vi "LabVIEW_ArduinoControlsNoHeater.vi"() -> ()   [LabVIEW 2021]
uses:
  <vilib>/Instr/_visa.llb/VISA Configure Serial Port (Instr).vi
panel:
  out "Horz Distance":dbl[](graph)
  out "Vert Distance":dbl[](graph)
  in  "DRILL STOP":bool
  in  "Drill Speed Arduino 2.0 Write Stop":bool
  in  "Slow Down":bool
  in  "Speed Up":bool
  in  "Drill Speed Arduino 2 Write":refnum<visa-resource-name>
  in  "Stepper Arduino 1 Serial Read":refnum<visa-resource-name>
  out "Weight on Bit A1":dbl[](graph)
  out "Vertical Motor Speed A1":dbl[](graph)
  out "Data Packet Arduini 1 Matched":i32
  in  "Arduino 1.0 Read Stop":bool
  in  "Arduino 2.0 Read Stop":bool
  in  "Emergency Stop! 3":bool
  in  "Emergency Stop! 2":bool
  in  "GO DOWN 3":bool
  in  "GO DOWN 2":bool
  in  "GO UP 3":bool
  in  "GO UP 2":bool
  in  "MAX SPEED 3":bool
  in  "MAX SPEED 2":bool
  in  "SLOWEST SPEED 3":bool
  in  "SLOWEST SPEED 2":bool
  in  "Decellerate 3":bool
  in  "Decellerate 2":bool
  in  "Accelerate 3":bool
  in  "Accelerate 2":bool
  in  "Drill Speed Arduino 2 Serial Read":refnum<visa-resource-name>
  out "Data Packet Received":i32
  out "RPM":dbl[](graph)
  in  "GO UP":bool
  in  "GO DOWN":bool
  in  "MAX SPEED":bool
  in  "SLOWEST SPEED":bool
  out "System Amps A2":dbl[](graph)
  out "concatenated string":string
  in  "Arduino 1.0 Write Stop":bool
  in  "Emergency Stop!":bool
  in  "Decellerate":bool
  in  "Stepper Arduino 1 Write":refnum<visa-resource-name>
  in  "Accelerate":bool
  # "Drill Speed Controls"
  # "WINCH CONTROLS"
  # "VERTICAL STEPPER MOTOR CONTROLS"
  # "HORIZONTAL STEPPER MOTOR CONTROLS"
  # "-1 Means Not Found\nany value greater than 0 corresponds to the amount\nof matching characters found"
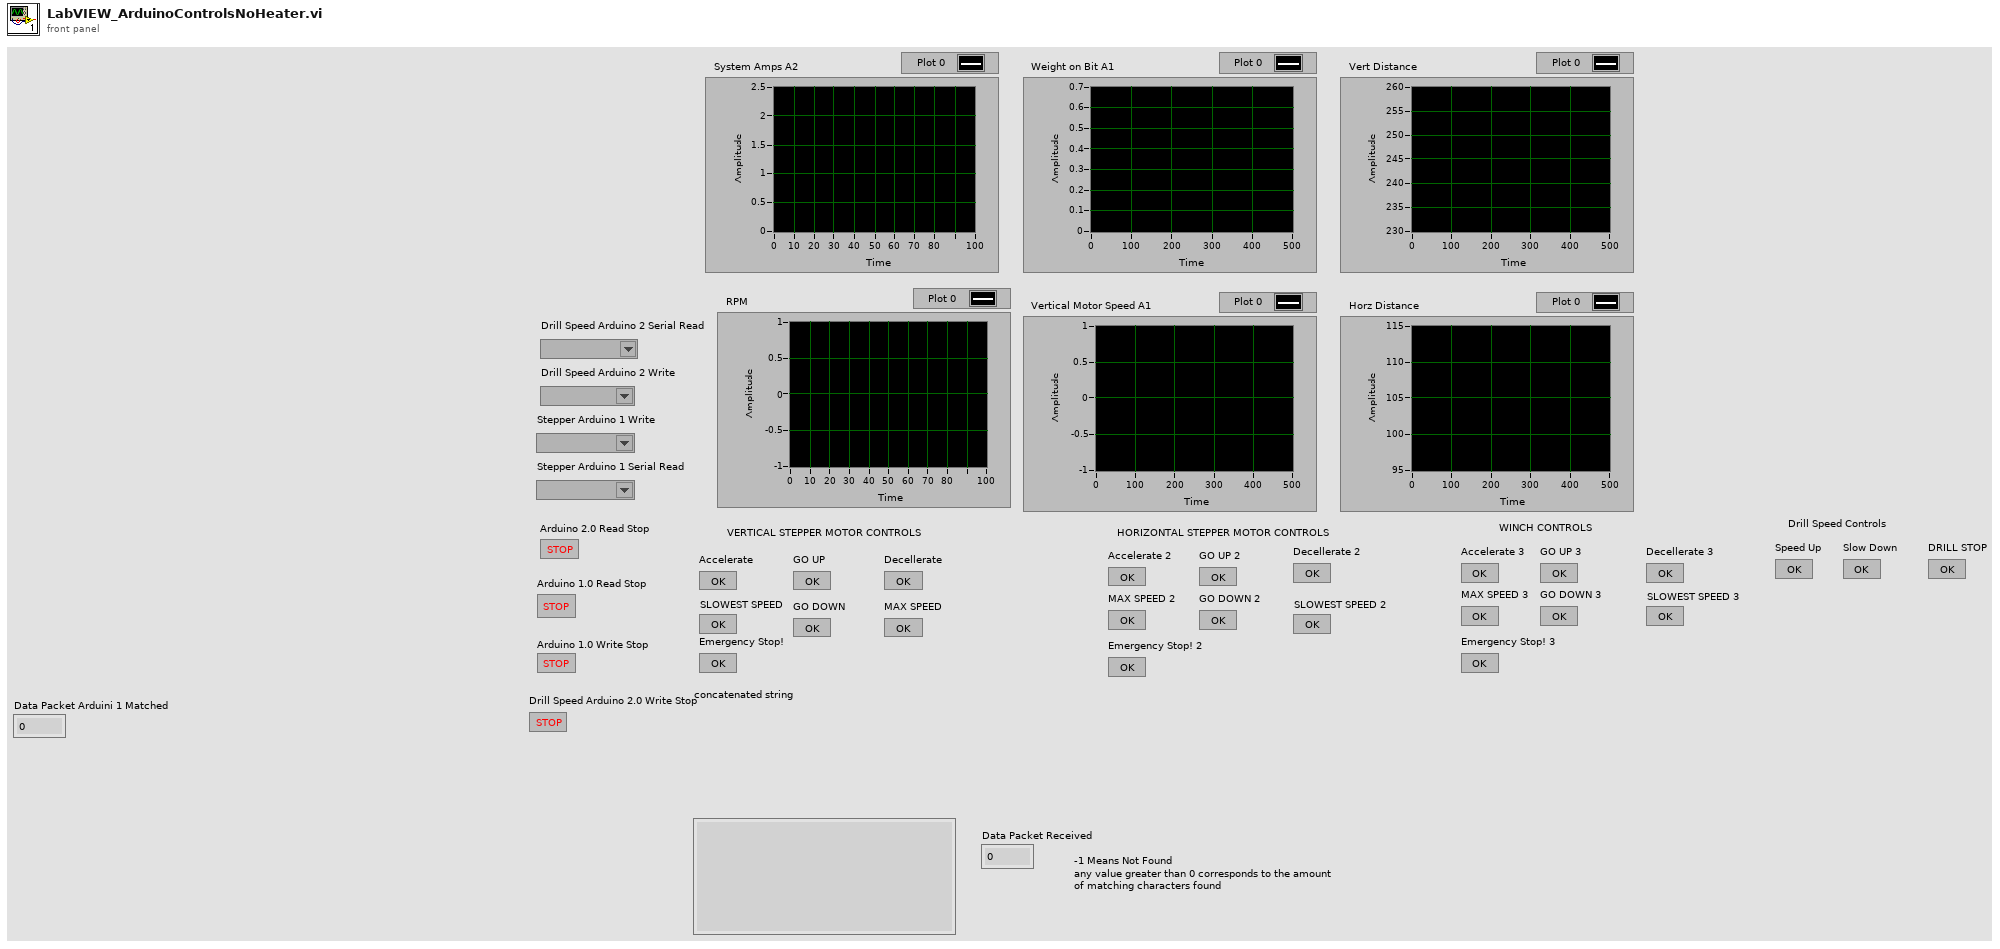
[diagram p1: front panel]
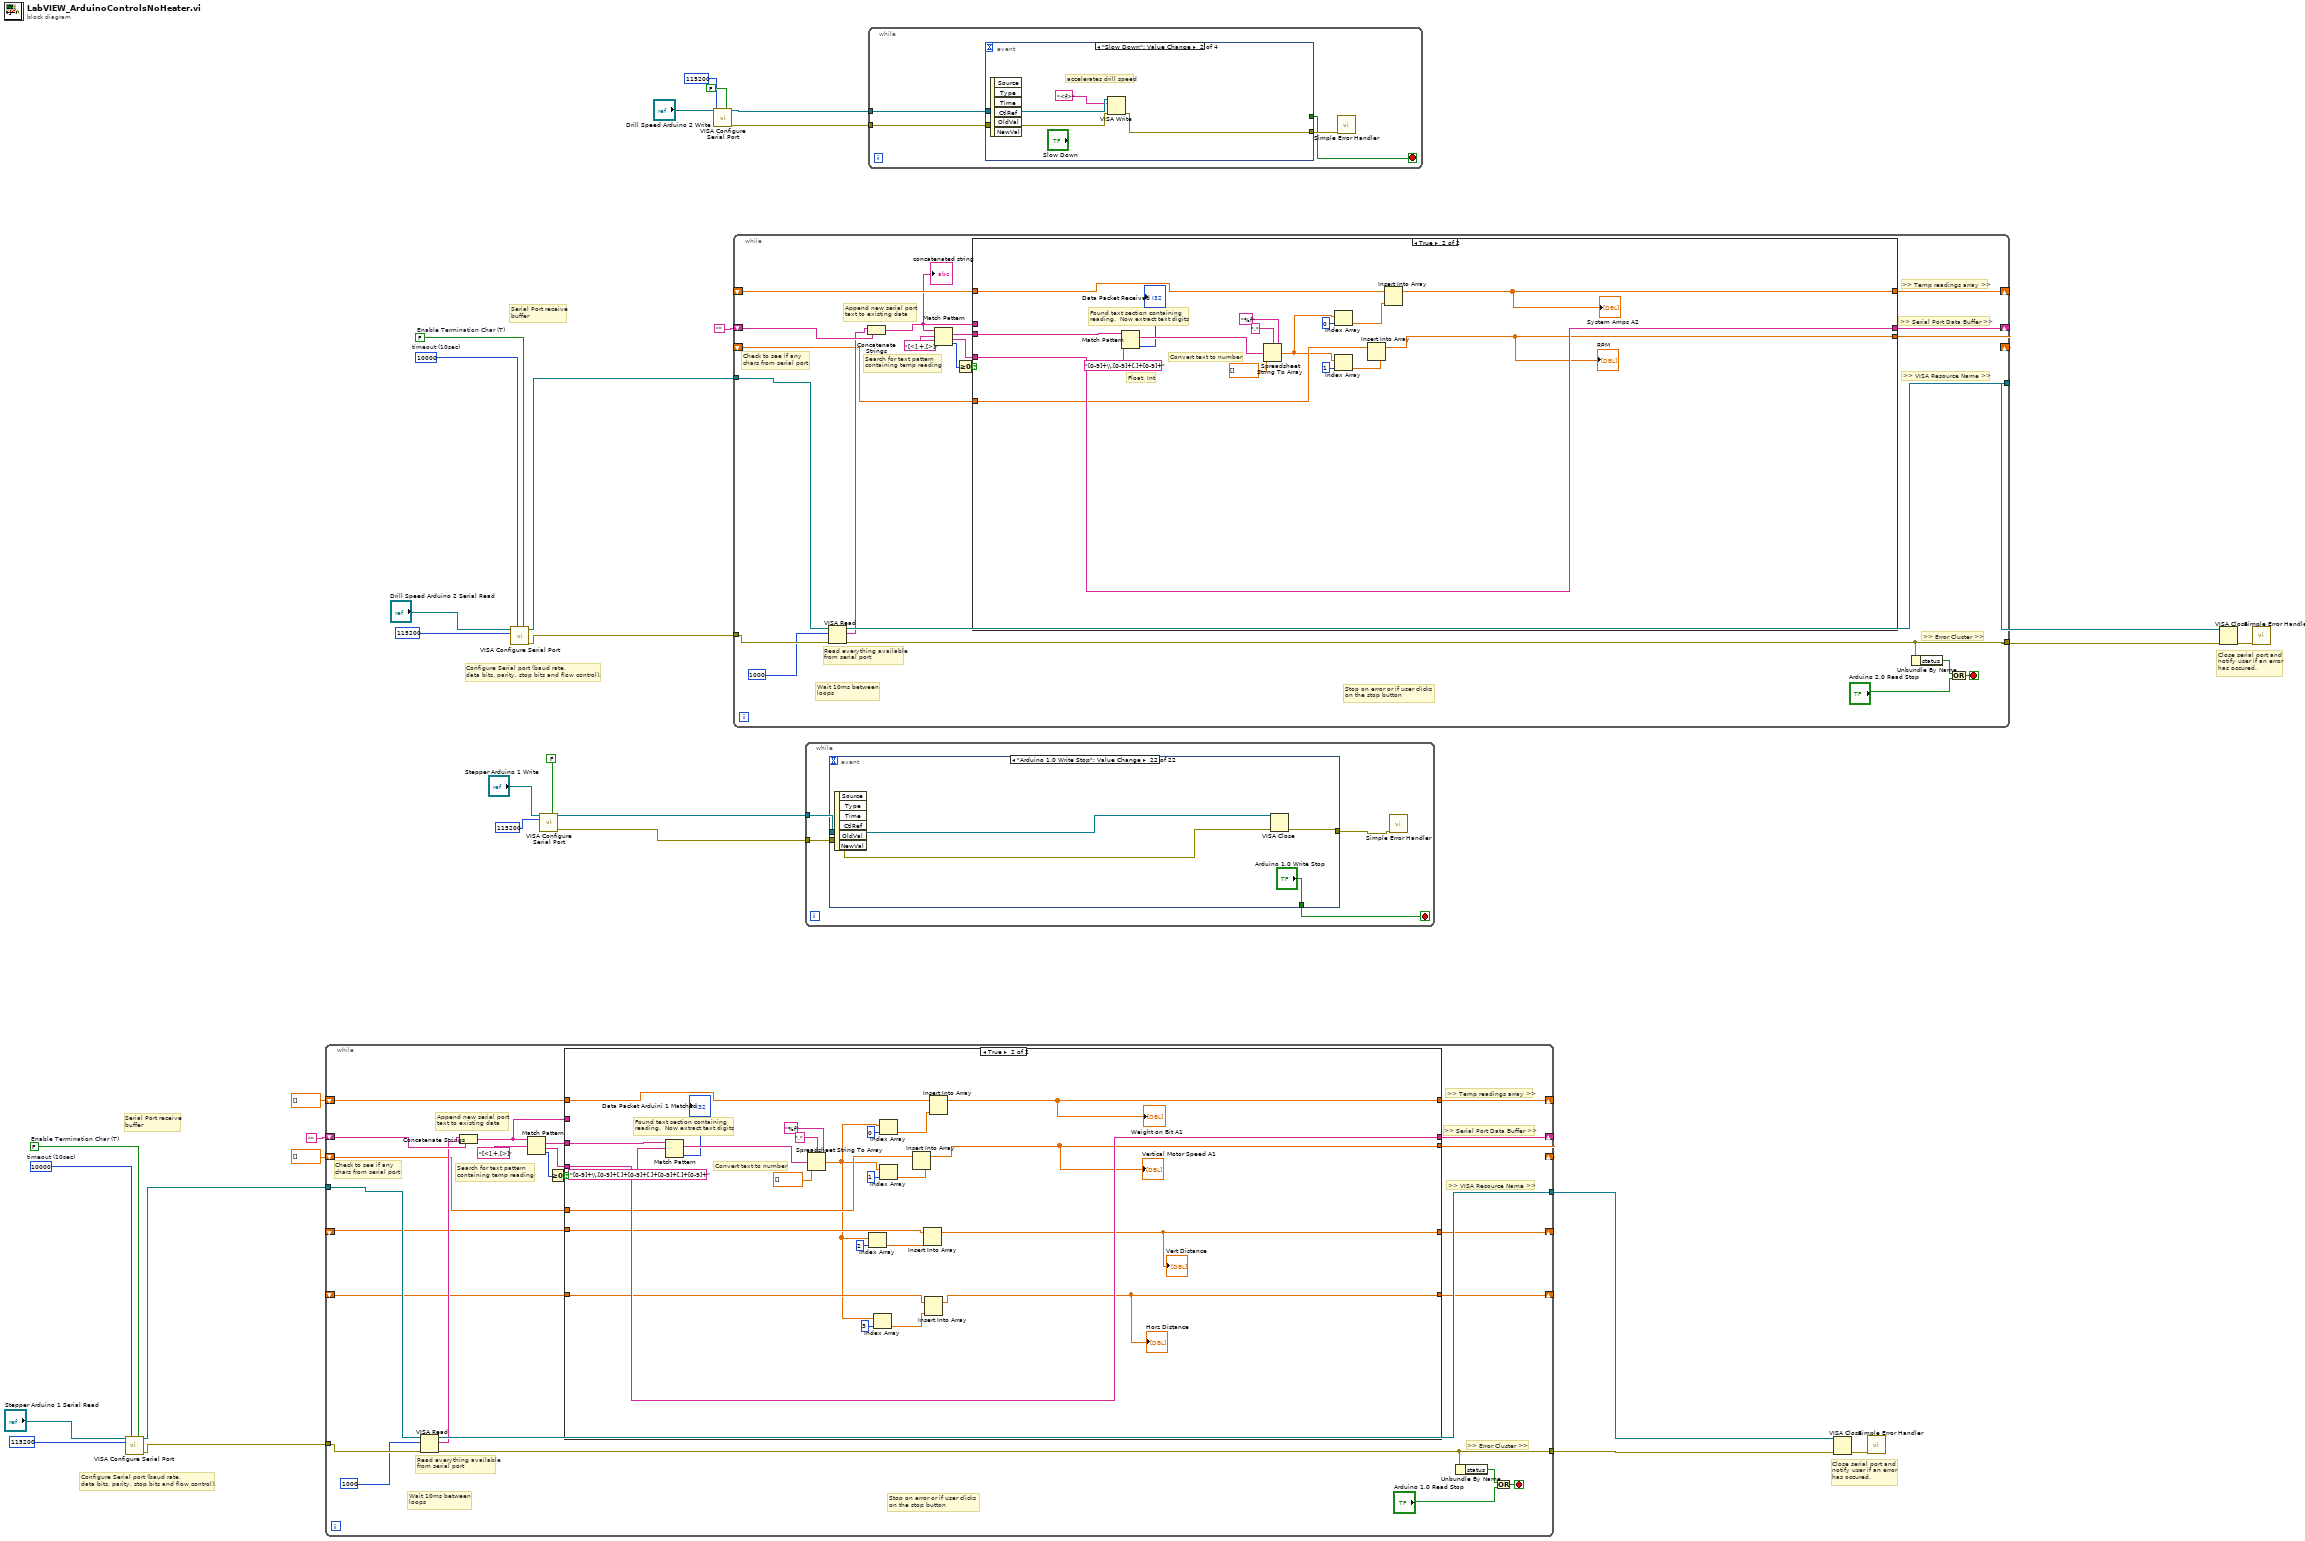
[diagram p0: block diagram]
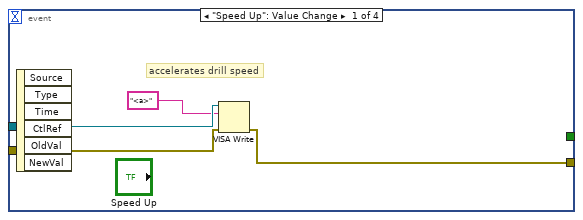
[diagram p2: hidden frame]
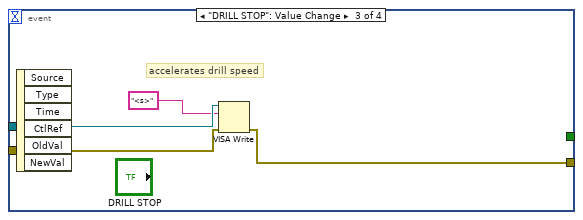
[diagram p3: hidden frame]
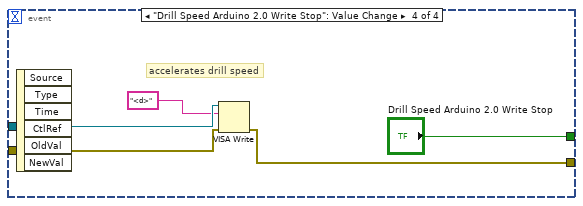
[diagram p4: hidden frame]
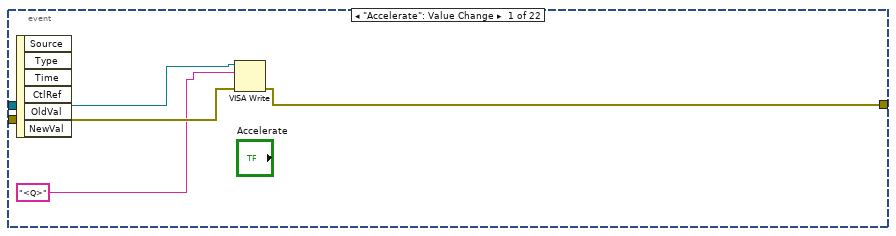
[diagram p7: hidden frame]
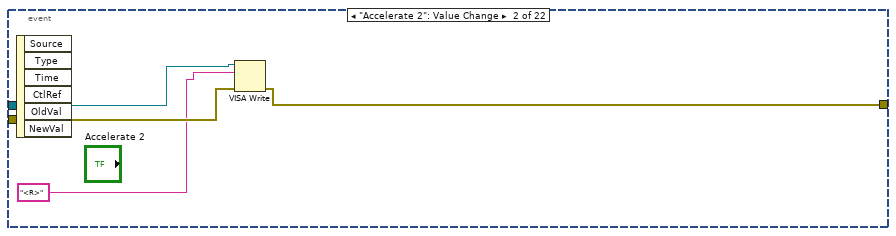
[diagram p8: hidden frame]
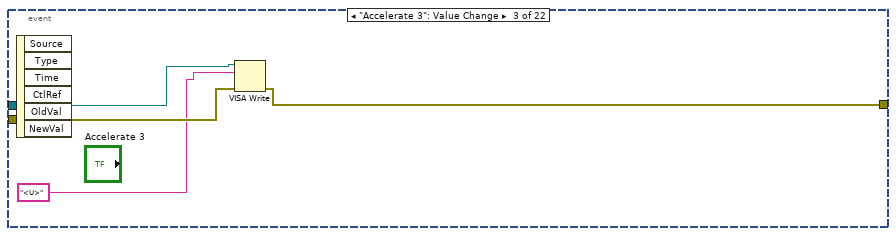
[diagram p9: hidden frame]
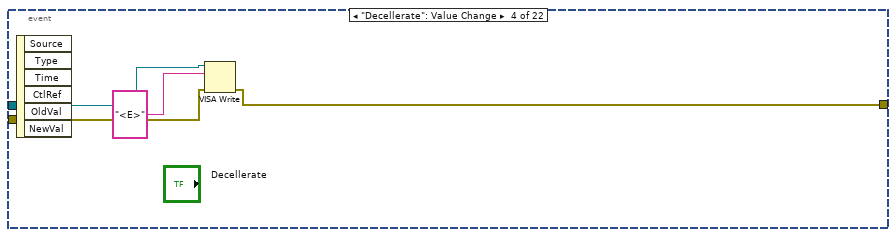
[diagram p10: hidden frame]
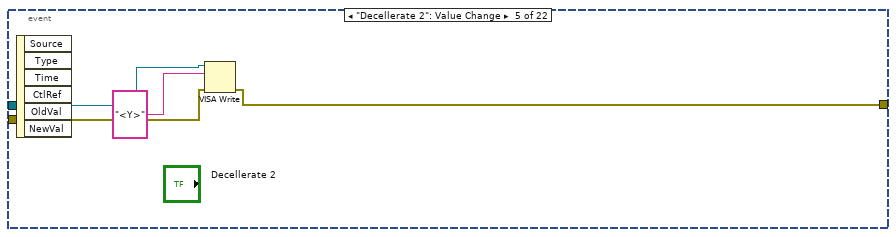
[diagram p11: hidden frame]
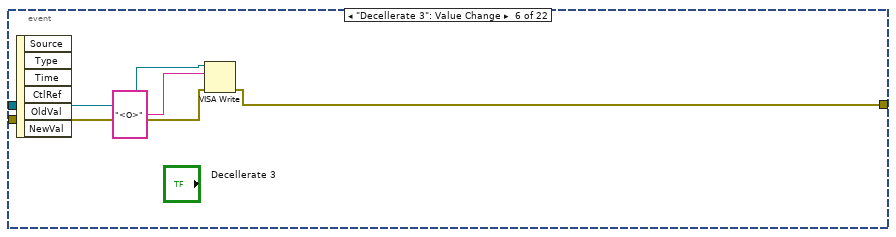
[diagram p12: hidden frame]
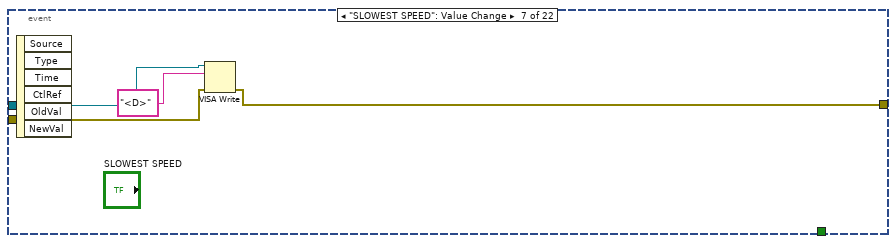
[diagram p13: hidden frame]
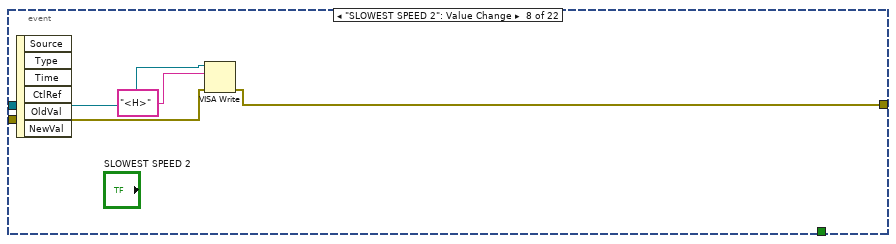
[diagram p14: hidden frame]
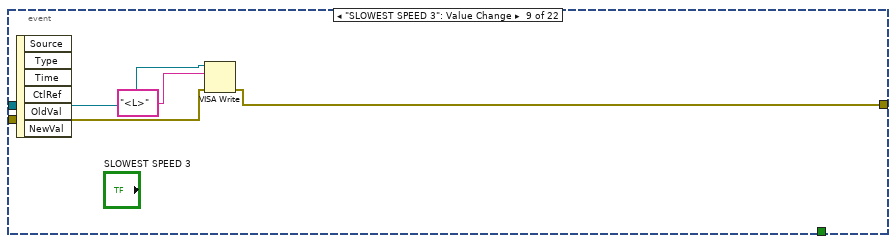
[diagram p15: hidden frame]
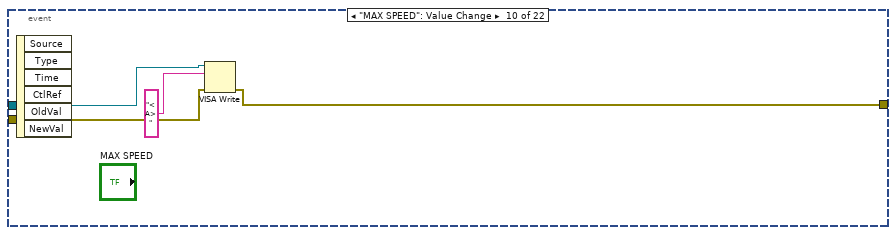
[diagram p16: hidden frame]
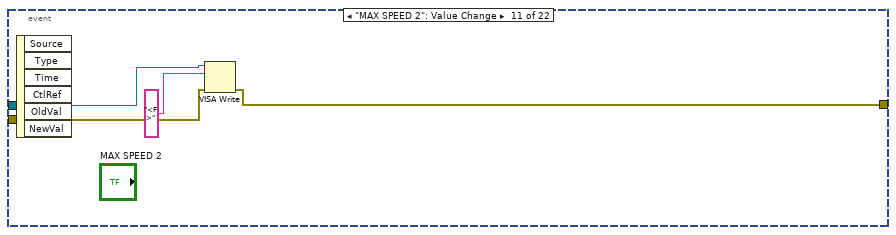
[diagram p17: hidden frame]
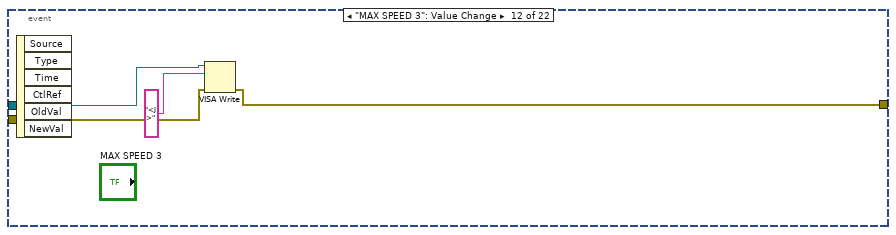
[diagram p18: hidden frame]
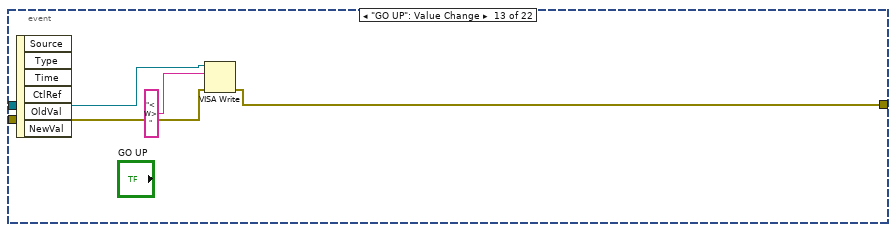
[diagram p19: hidden frame]
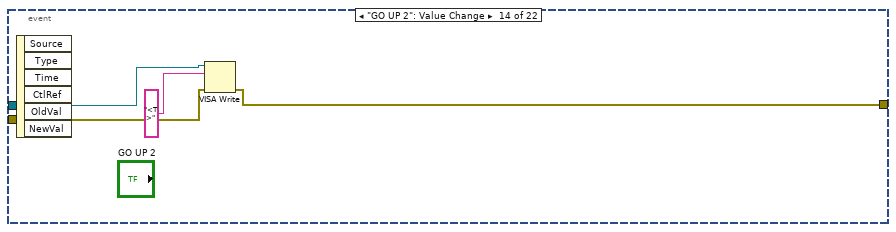
[diagram p20: hidden frame]
diagram:
  w13 = FALSE  # Enable Termination Char (T)
  w14 = u32 10000  # timeout (10sec)
  w24 = FALSE  # Enable Termination Char (T)
  w25 = u32 10000  # timeout (10sec)
  # "Close serial port and\nnotify user if an error\nhas occured."
  # "Serial Port receive\nbuffer"
  # "Configure Serial port (baud rate,\ndata bits, parity, stop bits and flow control)."
  # "Close serial port and\nnotify user if an error\nhas occured."
  # "Serial Port receive\nbuffer"
  # "Configure Serial port (baud rate,\ndata bits, parity, stop bits and flow control)."
  n1 = call-poly "VISA Configure Serial Port"("VISA resource name"="Stepper Arduino 1 Serial Read", "timeout (10sec)"=w14, "Enable Termination\nChar (T)"=w13, "baud rate (9600)"=u32 115200) -> ("VISA resource name out"=w10:refnum<visa-resource-name>, "error out"=w9:errorcluster)  [unwired: 10 in]
  n2 = while {
    tunnel: [w55] -> w17
    tunnel: [w57] -> w16
    shift-right: [w50] -> _
    shift-left: "" -> [w56]
    shift-right: [w52] -> _
    shift-left: dbl[] [] -> [w51]
    tunnel: w10 -> [w49]
    tunnel: w9 -> [w48]
    shift-right: [w40] -> _
    shift-left: dbl[] [] -> [w39]
    shift-right: [w35] -> _
    shift-left: _ -> [w36]
    shift-right: [w33] -> _
    shift-left: _ -> [w34]
    stop <- w54 stop-if-true
    # "Search for text pattern\ncontaining temp reading"
    # "Append new serial port\ntext to existing data"
    # "Read everything available\nfrom serial port"
    # "Wait 10ms between \nloops"
    # "Stop on error or if user clicks \non the stop button"
    # ">> Error Cluster >>"
    # ">> VISA Resource Name >>"
    # ">> Temp readings array >>"
    # ">> Serial Port Data Buffer >>"
    # "Check to see if any\nchars from serial port"
    n3 = VISA Read(VISA resource name=w49, byte count=u32 1000, error in (no error)=w48) -> (VISA resource name out=w57:refnum<visa-resource-name>, read buffer=w42:string, error out=w55:errorcluster)  [unwired: 1 out]
    n4 = Concatenate Strings(w42, w56) -> (w37:string)
    n5 = Match Pattern(string=w37, regular expression="[<].+.[>]") -> (match substring=w44:string, after substring=w43:string, offset past match=w46:i32)  [unwired: 1 in, 1 out]
    n6 = Greater Or Equal To 0?(x=w46) -> (x >= 0?=w45:bool)
    n7 = case shown="True" w45 {
      tunnel: w44 -> [_ w86]
      tunnel: w43 -> [_ w87]
      tunnel: [w60 w87] -> w50
      tunnel: [w62 w84] -> w52
      tunnel: w51 -> [w62 w72]
      tunnel: [w61 w75] -> w40
      tunnel: w39 -> [w61 w76]
      tunnel: w37 -> [w60 _]
      tunnel: w36 -> [w59 w70]
      tunnel: [w59 w68] -> w35
      tunnel: w34 -> [w58 w66]
      tunnel: [w58 w63] -> w33
      frame False {
        # "Did not find text pattern in the buffer.  Try again in the next loop after new data \nhas been received."
      }
      frame True {
        # "Convert text to number"
        # "Found text section containing \nreading.  Now extract text digits"
        n8 = Match Pattern(string=w86, regular expression="[0-9]+\\.[0-9]+[,]+[0-9]+[,]+[0-9]+[,]+[0-9]+") -> (match substring=w79:string, offset past match=→"Data Packet Arduini 1 Matched":i32)  [unwired: 1 in, 2 out]
        n9 = Spreadsheet String To Array(delimiter (Tab)=",", format string="%f", spreadsheet string=w79, array type (2D Dbl)=dbl[] []) -> (array=w65:dbl[])
        n10 = Index Array(array=w65, index=2) -> (element=w71:dbl)
        n11 = Index Array(array=w65, index=3) -> (element=w67:dbl)
        n12 = Index Array(array=w65, index=0 ("index (row)")) -> (element=w78:dbl)
        n13 = Index Array(array=w65, index=1 ("index (row)")) -> (element=w77:dbl)
        n14 = Insert Into Array(array=w76, new element=w77) -> (w75:dbl[])  [unwired: 1 in]
        "Vertical Motor Speed A1" <- w75
        n15 = Insert Into Array(array=w70, new element=w71) -> (w68:dbl[])  [unwired: 1 in]
        "Vert Distance" <- w68
        n16 = Insert Into Array(array=w66, new element=w67) -> (w63:dbl[])  [unwired: 1 in]
        "Horz Distance" <- w63
        n17 = Insert Into Array(array=w72, new element=w78) -> (w84:dbl[])  [unwired: 1 in]
        "Weight on Bit A1" <- w84
      }
    }
    n18 = Unbundle By Name(w55) -> ("status"=w53:bool)
    n19 = Or(x=w53, y="Arduino 1.0 Read Stop") -> (x .or. y?=w54:bool)
  }
  n20 = call-poly "VISA Configure Serial Port"("VISA resource name"="Drill Speed Arduino 2 Serial Read", "timeout (10sec)"=w25, "Enable Termination\nChar (T)"=w24, "baud rate (9600)"=u32 115200) -> ("VISA resource name out"=w21:refnum<visa-resource-name>, "error out"=w20:errorcluster)  [unwired: 10 in]
  n21 = call-poly "VISA Configure Serial Port"("VISA resource name"="Stepper Arduino 1 Write", "Enable Termination\nChar (T)"=FALSE ("Enable Termination\nChar (T)"), "baud rate (9600)"=u32 115200) -> ("VISA resource name out"=w32:refnum<visa-resource-name>, "error out"=w31:errorcluster)  [unwired: 11 in]
  n22 = call-poly "VISA Configure Serial Port"("VISA resource name"="Drill Speed Arduino 2 Write", "Enable Termination\nChar (T)"=FALSE ("Enable Termination\nChar (T)"), "baud rate (9600)"=u32 115200) -> ("VISA resource name out"=w7:refnum<visa-resource-name>, "error out"=w6:errorcluster)  [unwired: 11 in]
  n23 = while {
    tunnel: [w106] -> w28
    tunnel: [w108] -> w27
    shift-right: [w101] -> _
    shift-left: "" -> [w107]
    shift-right: [w103] -> _
    shift-left: _ -> [w102]
    tunnel: w21 -> [w100]
    tunnel: w20 -> [w99]
    shift-right: [w91] -> _
    shift-left: _ -> [w90]
    stop <- w105 stop-if-true
    # "Search for text pattern\ncontaining temp reading"
    # "Append new serial port\ntext to existing data"
    # "Read everything available\nfrom serial port"
    # "Wait 10ms between \nloops"
    # "Stop on error or if user clicks \non the stop button"
    # ">> Error Cluster >>"
    # ">> VISA Resource Name >>"
    # ">> Temp readings array >>"
    # ">> Serial Port Data Buffer >>"
    # "Check to see if any\nchars from serial port"
    n24 = VISA Read(VISA resource name=w100, byte count=u32 1000, error in (no error)=w99) -> (VISA resource name out=w108:refnum<visa-resource-name>, read buffer=w93:string, error out=w106:errorcluster)  [unwired: 1 out]
    n25 = Concatenate Strings(w93, w107) -> (w88:string)
    "concatenated string" <- w88
    n26 = Match Pattern(string=w88, regular expression="[<].+.[>]") -> (match substring=w95:string, after substring=w94:string, offset past match=w97:i32)  [unwired: 1 in, 1 out]
    n27 = Greater Or Equal To 0?(x=w97) -> (x >= 0?=w96:bool)
    n28 = case shown="True" w96 {
      tunnel: w95 -> [_ w127]
      tunnel: w94 -> [_ w128]
      tunnel: [w109 w128] -> w101
      tunnel: [w111 w125] -> w103
      tunnel: w102 -> [w111 w113]
      tunnel: [w110 w116] -> w91
      tunnel: w90 -> [w110 w117]
      tunnel: w88 -> [w109 _]
      frame False {
        # "Did not find text pattern in the buffer.  Try again in the next loop after new data \nhas been received."
      }
      frame True {
        # "Float, Int"
        # "Convert text to number"
        # "Found text section containing \nreading.  Now extract text digits"
        n29 = Match Pattern(string=w127, regular expression="[0-9]+\\.[0-9]+[,]+[0-9]+") -> (match substring=w120:string, offset past match=→"Data Packet Received":i32)  [unwired: 1 in, 2 out]
        n30 = Spreadsheet String To Array(delimiter (Tab)=",", format string="%f", spreadsheet string=w120, array type (2D Dbl)=dbl[] []) -> (array=w112:dbl[])
        n31 = Index Array(array=w112, index=0 ("index (row)")) -> (element=w119:dbl)
        n32 = Index Array(array=w112, index=1 ("index (row)")) -> (element=w118:dbl)
        n33 = Insert Into Array(array=w117, new element=w118) -> (w116:dbl[])  [unwired: 1 in]
        "RPM" <- w116
        n34 = Insert Into Array(array=w113, new element=w119) -> (w125:dbl[])  [unwired: 1 in]
        "System Amps A2" <- w125
      }
    }
    n35 = Unbundle By Name(w106) -> ("status"=w104:bool)
    n36 = Or(x=w104, y="Arduino 2.0 Read Stop") -> (x .or. y?=w105:bool)
  }
  n37 = while {
    tunnel: w32 -> [w132]
    tunnel: w31 -> [w131]
    stop <- w129 stop-if-true
    n38 = event shown="[21] \"Arduino 1.0 Write Stop\": Value Change" {
      selector: _ -> [_ _ _ _ _ _ _ _ _ _ _ _ _ _ _ _ _ _ _ _ _ _]
      dyn-events: _ -> [_ _ _ _ _ _ _ _ _ _ _ _ _ _ _ _ _ _ _ _ _ _]
      timeout: _ -> [_ _ _ _ _ _ _ _ _ _ _ _ _ _ _ _ _ _ _ _ _ _]
      tunnel: [w136 w140 w144 w148 w152 w156 w160 w164 w168 w172 w176 w180 w184 w188 w192 w196 w200 w204 w208 w212 w216 w220] -> w130
      tunnel: w132 -> [w135 w139 w143 w146 w150 w154 w158 w162 w166 w170 w174 w178 w182 w186 w190 w194 w198 w202 w206 w210 w214 w219]
      tunnel: w131 -> [w134 w138 w142 w145 w149 w153 w157 w161 w165 w169 w173 w177 w181 w185 w189 w193 w197 w201 w205 w209 w213 w218]
      tunnel: [_ _ _ _ _ _ _ _ _ _ _ _ _ _ _ _ _ _ _ _ _ "Arduino 1.0 Write Stop"] -> w129
      event "Accelerate": Value Change {
        n39 = event-data() -> ()  [unwired: 1 in, 6 out]
        n40 = VISA Write(VISA resource name=w135, write buffer="<Q>", error in (no error)=w134) -> (error out=w136:errorcluster)  [unwired: 2 out]
      }
      event "Accelerate 2": Value Change {
        n41 = event-data() -> ()  [unwired: 1 in, 6 out]
        n42 = VISA Write(VISA resource name=w139, write buffer="<R>", error in (no error)=w138) -> (error out=w140:errorcluster)  [unwired: 2 out]
      }
      event "Accelerate 3": Value Change {
        n43 = event-data() -> ()  [unwired: 1 in, 6 out]
        n44 = VISA Write(VISA resource name=w143, write buffer="<U>", error in (no error)=w142) -> (error out=w144:errorcluster)  [unwired: 2 out]
      }
      event "Decellerate": Value Change {
        n45 = event-data() -> ()  [unwired: 1 in, 6 out]
        n46 = VISA Write(VISA resource name=w146, write buffer="<E>", error in (no error)=w145) -> (error out=w148:errorcluster)  [unwired: 2 out]
      }
      event "Decellerate 2": Value Change {
        n47 = event-data() -> ()  [unwired: 1 in, 6 out]
        n48 = VISA Write(VISA resource name=w150, write buffer="<Y>", error in (no error)=w149) -> (error out=w152:errorcluster)  [unwired: 2 out]
      }
      event "Decellerate 3": Value Change {
        n49 = event-data() -> ()  [unwired: 1 in, 6 out]
        n50 = VISA Write(VISA resource name=w154, write buffer="<O>", error in (no error)=w153) -> (error out=w156:errorcluster)  [unwired: 2 out]
      }
      event "SLOWEST SPEED": Value Change {
        n51 = event-data() -> ()  [unwired: 1 in, 6 out]
        n52 = VISA Write(VISA resource name=w158, write buffer="<D>", error in (no error)=w157) -> (error out=w160:errorcluster)  [unwired: 2 out]
      }
      event "SLOWEST SPEED 2": Value Change {
        n53 = event-data() -> ()  [unwired: 1 in, 6 out]
        n54 = VISA Write(VISA resource name=w162, write buffer="<H>", error in (no error)=w161) -> (error out=w164:errorcluster)  [unwired: 2 out]
      }
      event "SLOWEST SPEED 3": Value Change {
        n55 = event-data() -> ()  [unwired: 1 in, 6 out]
        n56 = VISA Write(VISA resource name=w166, write buffer="<L>", error in (no error)=w165) -> (error out=w168:errorcluster)  [unwired: 2 out]
      }
      event "MAX SPEED": Value Change {
        n57 = event-data() -> ()  [unwired: 1 in, 6 out]
        n58 = VISA Write(VISA resource name=w170, write buffer="<A>", error in (no error)=w169) -> (error out=w172:errorcluster)  [unwired: 2 out]
      }
      event "MAX SPEED 2": Value Change {
        n59 = event-data() -> ()  [unwired: 1 in, 6 out]
        n60 = VISA Write(VISA resource name=w174, write buffer="<F>", error in (no error)=w173) -> (error out=w176:errorcluster)  [unwired: 2 out]
      }
      event "MAX SPEED 3": Value Change {
        n61 = event-data() -> ()  [unwired: 1 in, 6 out]
        n62 = VISA Write(VISA resource name=w178, write buffer="<J>", error in (no error)=w177) -> (error out=w180:errorcluster)  [unwired: 2 out]
      }
      event "GO UP": Value Change {
        n63 = event-data() -> ()  [unwired: 1 in, 6 out]
        n64 = VISA Write(VISA resource name=w182, write buffer="<W>", error in (no error)=w181) -> (error out=w184:errorcluster)  [unwired: 2 out]
      }
      event "GO UP 2": Value Change {
        n65 = event-data() -> ()  [unwired: 1 in, 6 out]
        n66 = VISA Write(VISA resource name=w186, write buffer="<T>", error in (no error)=w185) -> (error out=w188:errorcluster)  [unwired: 2 out]
      }
      event "GO UP 3": Value Change {
        n67 = event-data() -> ()  [unwired: 1 in, 6 out]
        n68 = VISA Write(VISA resource name=w190, write buffer="<I>", error in (no error)=w189) -> (error out=w192:errorcluster)  [unwired: 2 out]
      }
      event "GO DOWN": Value Change {
        n69 = event-data() -> ()  [unwired: 1 in, 6 out]
        n70 = VISA Write(VISA resource name=w194, write buffer="<S>", error in (no error)=w193) -> (error out=w196:errorcluster)  [unwired: 2 out]
      }
      event "GO DOWN 2": Value Change {
        n71 = event-data() -> ()  [unwired: 1 in, 6 out]
        n72 = VISA Write(VISA resource name=w198, write buffer="<G>", error in (no error)=w197) -> (error out=w200:errorcluster)  [unwired: 2 out]
      }
      event "GO DOWN 3": Value Change {
        n73 = event-data() -> ()  [unwired: 1 in, 6 out]
        n74 = VISA Write(VISA resource name=w202, write buffer="<K>", error in (no error)=w201) -> (error out=w204:errorcluster)  [unwired: 2 out]
      }
      event "Emergency Stop!": Value Change {
        n75 = event-data() -> ()  [unwired: 1 in, 6 out]
        n76 = VISA Write(VISA resource name=w206, write buffer="<Z>", error in (no error)=w205) -> (error out=w208:errorcluster)  [unwired: 2 out]
      }
      event "Emergency Stop! 2": Value Change {
        n77 = event-data() -> ()  [unwired: 1 in, 6 out]
        n78 = VISA Write(VISA resource name=w210, write buffer="<C>", error in (no error)=w209) -> (error out=w212:errorcluster)  [unwired: 2 out]
      }
      event "Emergency Stop! 3": Value Change {
        n79 = event-data() -> ()  [unwired: 1 in, 6 out]
        n80 = VISA Write(VISA resource name=w214, write buffer="<N>", error in (no error)=w213) -> (error out=w216:errorcluster)  [unwired: 2 out]
      }
      event "Arduino 1.0 Write Stop": Value Change {
        n81 = event-data() -> ()  [unwired: 1 in, 6 out]
        n82 = VISA Close(VISA resource name=w219, error in (no error)=w218) -> (error out=w220:errorcluster)
      }
    }
    n83 = call <vilib>:"Simple Error Handler.vi"("error in (no error)"=w130) -> ()  [unwired: 4 in, 5 out]
  }
  n84 = while {
    tunnel: w7 -> [w224]
    tunnel: w6 -> [w223]
    stop <- w221 stop-if-true
    n85 = event shown="[1] \"Slow Down\": Value Change" {
      selector: _ -> [_ _ _ _]
      dyn-events: _ -> [_ _ _ _]
      timeout: _ -> [_ _ _ _]
      tunnel: w224 -> [w228 w232 w236 w241]
      tunnel: w223 -> [w227 w231 w235 w240]
      tunnel: [w225 w229 w233 w238] -> w222
      tunnel: [_ _ _ "Drill Speed Arduino 2.0 Write Stop"] -> w221
      event "Speed Up": Value Change {
        # "accelerates drill speed"
        n86 = event-data() -> ()  [unwired: 1 in, 6 out]
        n87 = VISA Write(VISA resource name=w228, write buffer="<a>", error in (no error)=w227) -> (error out=w225:errorcluster)  [unwired: 2 out]
      }
      event "Slow Down": Value Change {
        # "accelerates drill speed"
        n88 = event-data() -> ()  [unwired: 1 in, 6 out]
        n89 = VISA Write(VISA resource name=w232, write buffer="<f>", error in (no error)=w231) -> (error out=w229:errorcluster)  [unwired: 2 out]
      }
      event "DRILL STOP": Value Change {
        # "accelerates drill speed"
        n90 = event-data() -> ()  [unwired: 1 in, 6 out]
        n91 = VISA Write(VISA resource name=w236, write buffer="<s>", error in (no error)=w235) -> (error out=w233:errorcluster)  [unwired: 2 out]
      }
      event "Drill Speed Arduino 2.0 Write Stop": Value Change {
        # "accelerates drill speed"
        n92 = event-data() -> ()  [unwired: 1 in, 6 out]
        n93 = VISA Write(VISA resource name=w241, write buffer="<d>", error in (no error)=w240) -> (error out=w238:errorcluster)  [unwired: 2 out]
      }
    }
    n94 = call <vilib>:"Simple Error Handler.vi"("error in (no error)"=w222) -> ()  [unwired: 4 in, 5 out]
  }
  n95 = VISA Close(VISA resource name=w16, error in (no error)=w17) -> (error out=w15:errorcluster)
  n96 = call <vilib>:"Simple Error Handler.vi"("error in (no error)"=w15) -> ()  [unwired: 4 in, 5 out]
  n97 = VISA Close(VISA resource name=w27, error in (no error)=w28) -> (error out=w26:errorcluster)
  n98 = call <vilib>:"Simple Error Handler.vi"("error in (no error)"=w26) -> ()  [unwired: 4 in, 5 out]
